vi "RecordSectionIMAQdx.vi"() -> ()   [LabVIEW 2009]
doc: "The Grab VI acquires images continuously and displays the images in an image control using high-level acquisition VIs. A grab is appropriate for high-speed applications in which you need to process only one image at a time."
uses:
  <vilib>/vision/driver/NI_Vision_Acquisition_Software.lvlib
  <vilib>/vision/Avi.llb/IMAQ AVI2 Refnum.ctl
panel:
  in  "Camera Name":refnum<k21> caption="IMAQdx Session"
  in  "Stop":bool
  out "Image":T1(plugin-control)
  in  "AVI File Path":path
  in  "Record":bool
  # "Overview: Demonstrates how to record a section of video while continuously using a Grab acquisition.  Can start and stop recording to specified AVI file path.\nRequirements: Vision Acquisition Software\nInstructions: \n1. Specify AVI File Path\n2. Select the Camera Interface.\n3. Run the VI\n4. Set Record booelean to true during segment of Grab you wish to record to AVI\n5. Set Recor boolean to false to end recording.\n6. Click Stop to terminate program."
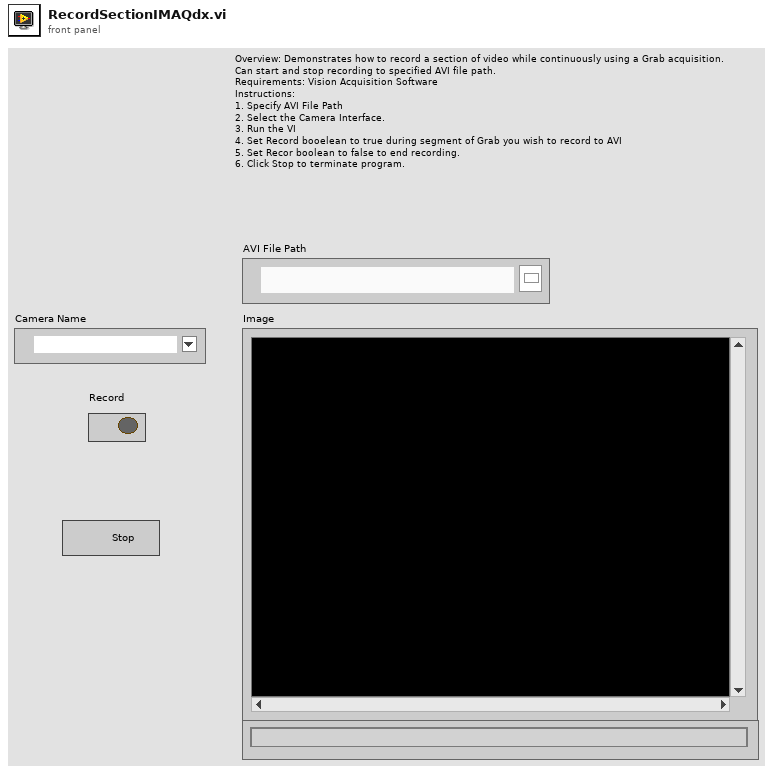
[diagram p1: front panel]
types:
  T1 = typedef "IMAQ Image.ctl" = refnum<image>
  T2 = typedef "Image Type" = u32
  T3 = typedef "IMAQdx.ctl" = refnum<k21>
  T4 = typedef "IMAQ AVI2 Refnum.ctl" = refnum<k20>
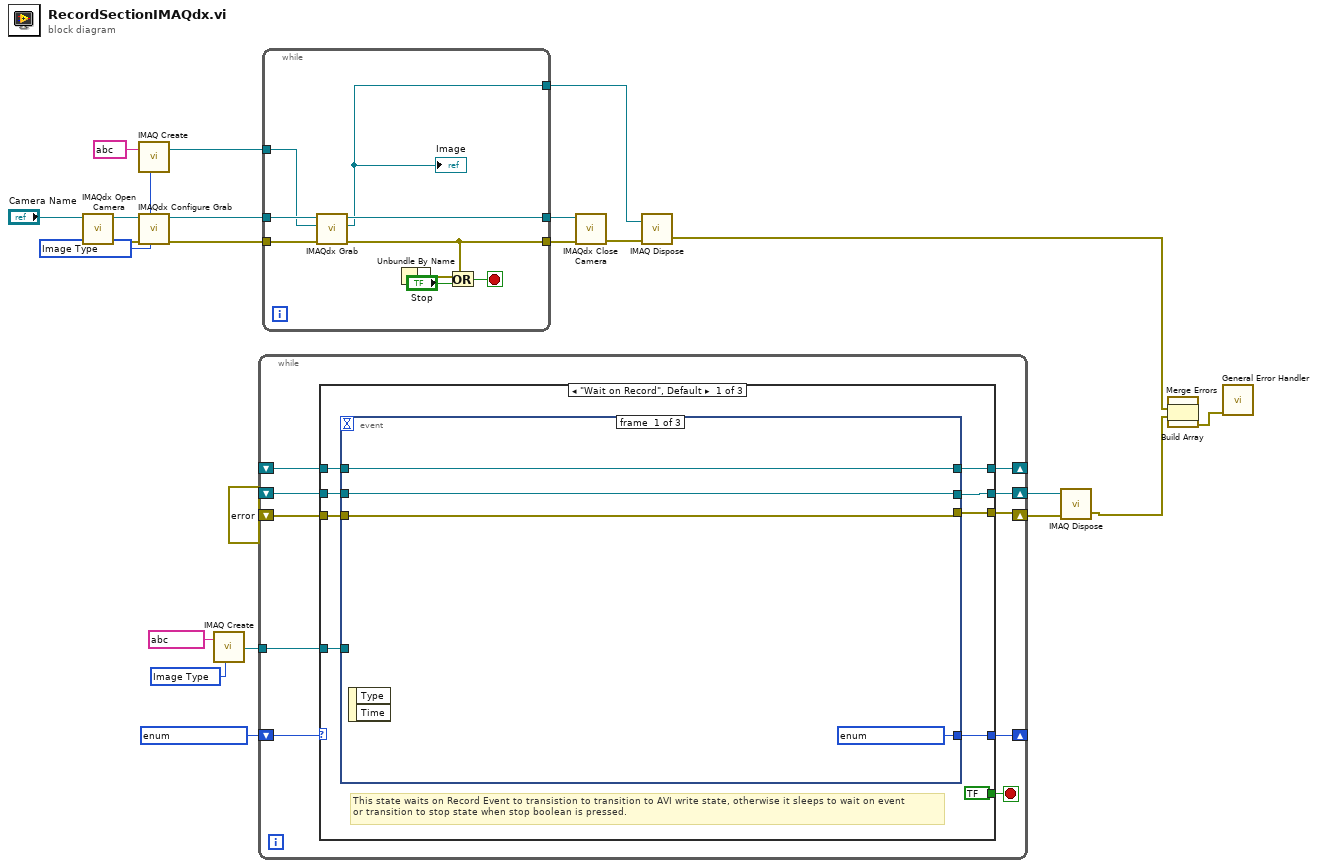
[diagram p0: block diagram]
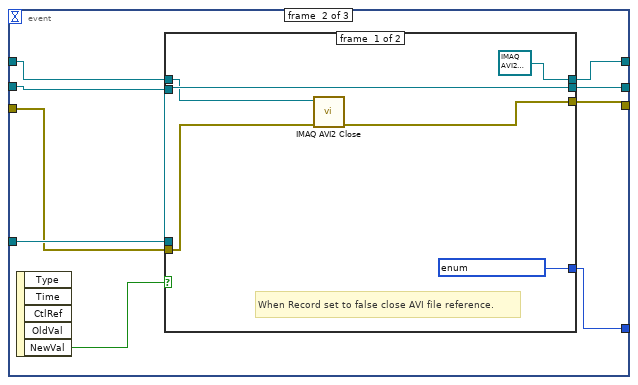
[diagram p2: hidden frame]
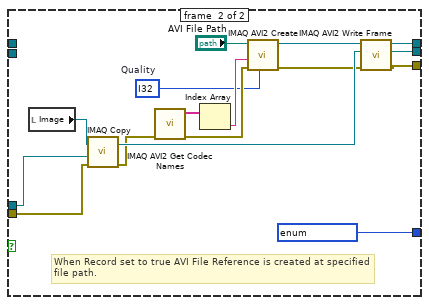
[diagram p3: hidden frame]
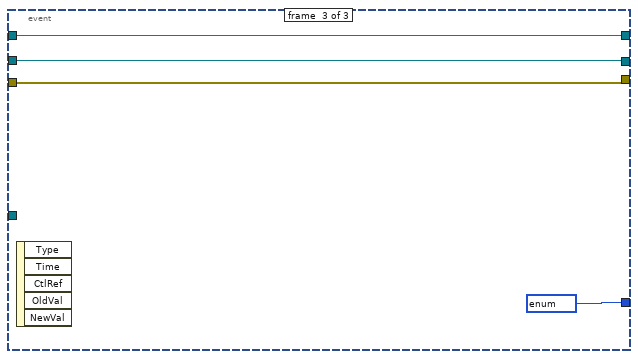
[diagram p4: hidden frame]
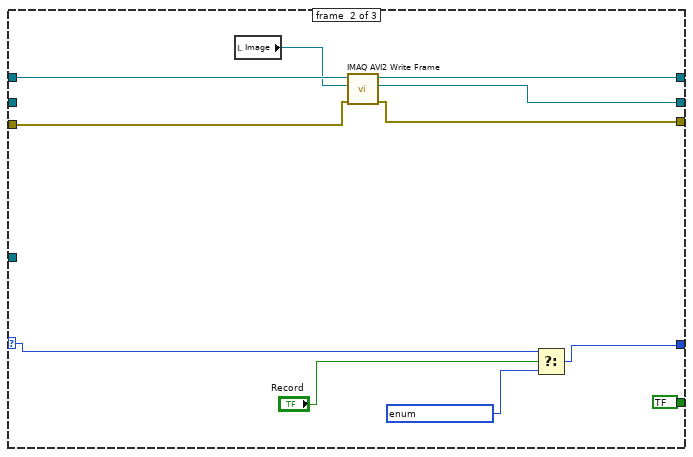
[diagram p5: hidden frame]
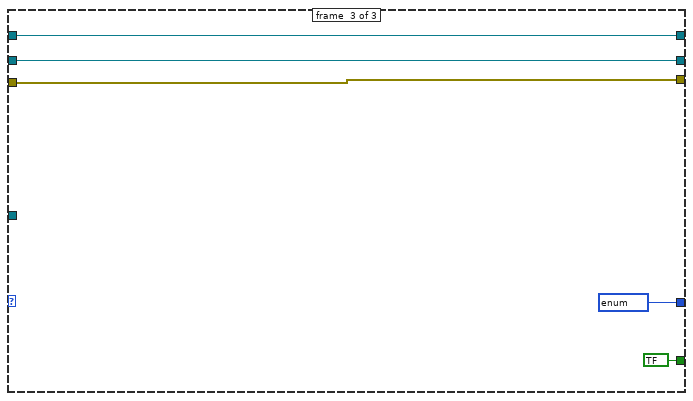
[diagram p6: hidden frame]
diagram:
  w2 = T2 ? items=["Grayscale (U8)", "Grayscale (I16)", "Grayscale (SGL)", "Complex (CSG)", "RGB (U32)", "HSL (U32)", "RGB (U64)", "Grayscale (U16)"] ("Image Type")
  w19 = T2 ? items=["Grayscale (U8)", "Grayscale (I16)", "Grayscale (SGL)", "Complex (CSG)", "RGB (U32)", "HSL (U32)", "RGB (U64)", "Grayscale (U16)"] ("Image Type")
  n1 = call <vilib>:"IMAQdx Open Camera.vi"("Session In"="Camera Name") -> ("error out"=w10:errorcluster, "Session Out"=w9:T3)  [unwired: 2 in, 7 out]
  n2 = call "IMAQ Create"("Image Name"=string ?, "Image Type"=w2) -> ("New Image"=w15:T1)  [unwired: 2 in, 2 out]
  n3 = call <vilib>:"IMAQdx Configure Grab.vi"("error in"=w10, "Session In"=w9) -> ("error out"=w13:errorcluster, "Session Out"=w14:T3)  [unwired: 8 out]
  n4 = call "IMAQ Create"("Image Name"=string ?, "Image Type"=w19) -> ("New Image"=w22:T1)  [unwired: 3 in, 1 out]
  n5 = while {
    tunnel: w22 -> [w33]
    shift-right: [w29] -> _
    shift-left: enum16{"Wait on Record", "Recording", "Stop"} ? -> [w30]
    shift-right: [w28] -> _
    shift-left: _ -> [w27]
    shift-right: [w31] -> w20
    shift-left: errorcluster ? ("error out") -> [w26]
    shift-right: [w32] -> w21
    shift-left: _ -> [w24]
    stop <- w25 stop-if-true
    n6 = case shown="\"Wait on Record\", Default" w30 {
      selector: w30 -> [_ w82 _]
      tunnel: w33 -> [w42 _ _]
      tunnel: [w41 w85 w93] -> w32
      tunnel: [w40 w88 w95] -> w31
      tunnel: [w39 w87 enum16{"Wait on Record", "Recording", "Stop"} ?] -> w29
      tunnel: [w38 w91 w96] -> w28
      tunnel: w27 -> [w37 w92 w96]
      tunnel: w26 -> [w36 w89 w95]
      tunnel: [bool ? bool ? bool ?] -> w25
      tunnel: w24 -> [w34 _ w93]
      frame #0 {
        # "This state waits on Record Event to transistion to transition to AVI write state, otherwise it sleeps to wait on event\nor transition to stop state when stop boolean is pressed."
        n7 = event shown="[1] \"Record\": Value Change" {
          selector: _ -> [_ _ _]
          dyn-events: _ -> [_ _ _]
          timeout: _ -> [_ _ _]
          tunnel: w42 -> [_ w55 _]
          tunnel: [w45 w54 w79] -> w41
          tunnel: [w46 w53 w78] -> w40
          tunnel: [enum16{"Wait on Record", "Recording", "Stop"} ? w47 enum16{"Wait on Record", "Recording", "Stop"} ?] -> w39
          tunnel: [w44 w52 w80] -> w38
          tunnel: w37 -> [w44 w50 w80]
          tunnel: w36 -> [w46 w51 w78]
          tunnel: w34 -> [w45 w49 w79]
          event #0 {
            n8 = event-data() -> ()  [unwired: 1 in, 2 out]
          }
          event #1 {
            n9 = event-data() -> ("NewVal"=w48:bool)  [unwired: 1 in, 4 out]
            n10 = case shown="True" w48 {
              tunnel: w55 -> [w61 w77]
              tunnel: [w61 w70] -> w54
              tunnel: [w57 w69] -> w53
              tunnel: [T4 ? ("AVI Refnum (duplicate)") w66] -> w52
              tunnel: w51 -> [w58 w63]
              tunnel: w50 -> [w59 _]
              tunnel: w49 -> [_ _]
              tunnel: [enum16{"Wait on Record", "Recording", "Stop"} ? enum16{"Wait on Record", "Recording", "Stop"} ?] -> w47
              frame #0 {
                # "When Record set to false close AVI file reference."
                n11 = call "IMAQ AVI2 Close"("error in (no error)"=w58, "AVI Refnum"=w59) -> ("error out"=w57:errorcluster)  [unwired: 9 in]
              }
              frame #1 {
                w73 = i32 ?  # Quality
                # "When Record set to true AVI File Reference is created at specified file path."
                n12 = local read "Image"() -> (w76:T1)
                n13 = call "IMAQ Copy"("error in (no error)"=w63, "Image Dst"=w77, "Image Src"=w76) -> ("error out"=w64:errorcluster, "Image Dst Out"=w68:T1)  [unwired: 3 in]
                n14 = call "IMAQ AVI2 Get Codec Names"("error in (no error)"=w64) -> ("error out"=w75:errorcluster, "Codec Names"=w72:string[])  [unwired: 9 in]
                n15 = Index Array(array=w72) -> (element=w74:string)  [unwired: 1 in]
                n16 = call "IMAQ AVI2 Create"("Quality"=w73, "error in (no error)"=w75, "Codec"=w74, "AVI Path"="AVI File Path") -> ("error out"=w65:errorcluster, "AVI Refnum"=w67:T4)  [unwired: 6 in]
                n17 = call "IMAQ AVI2 Write Frame"("error in (no error)"=w65, "Image"=w68, "AVI Refnum"=w67) -> ("error out"=w69:errorcluster, "Image Out (duplicate)"=w70:T1, "AVI Refnum (duplicate)"=w66:T4)  [unwired: 6 in]
              }
            }
          }
          event #2 {
            n18 = event-data() -> ()  [unwired: 1 in, 5 out]
          }
        }
      }
      frame #1 {
        n19 = local read "Image"() -> (w90:T1)
        n20 = call "IMAQ AVI2 Write Frame"("error in (no error)"=w89, "Image"=w90, "AVI Refnum"=w92) -> ("error out"=w88:errorcluster, "Image Out (duplicate)"=w85:T1, "AVI Refnum (duplicate)"=w91:T4)  [unwired: 6 in]
        n21 = Select(t=w82, s="Record", f=enum16{"Wait on Record", "Recording", "Stop"} ?) -> (s? t:f=w87:enum16{"Wait on Record", "Recording", "Stop"})
      }
      frame #2 {
      }
    }
  }
  n22 = while {
    tunnel: [w101] -> w12
    tunnel: w13 -> [w103]
    tunnel: w14 -> [w104]
    tunnel: [w100] -> w11
    tunnel: w15 -> [w102]
    tunnel: [w99] -> w7
    stop <- w106 stop-if-true
    n23 = call <vilib>:"IMAQdx Grab.vi"("error in"=w103, "Image In"=w102, "Session In"=w104) -> ("error out"=w100:errorcluster, "Image Out"=w99:T1, "Session Out"=w101:T3)  [unwired: 1 in, 5 out]
    "Image" <- w99
    n24 = Or(y="Stop") -> (x=w98:errorcluster, x .or. y?=w106:bool)
    n25 = Unbundle By Name(w100, w98) -> ()
  }
  n26 = call <vilib>:"IMAQdx Close Camera.vi"("error in"=w11, "Session In"=w12) -> ("error out"=w6:errorcluster)  [unwired: 9 out]
  n27 = call "IMAQ Dispose"("Image"=w7, "error in (no error)"=w6) -> ("error out"=w4:errorcluster)  [unwired: 4 in]
  n28 = call "IMAQ Dispose"("Image"=w21, "error in (no error)"=w20) -> ("error out"=w3:errorcluster)  [unwired: 1 in, 3 out]
  n29 = Build Array(w4, w3) -> (w1:errorcluster[])
  n30 = call <vilib>:"Merge Errors.vi"("error array in"=w1) -> ("error out"=w17:errorcluster)  [unwired: 6 in]
  n31 = call <vilib>:"General Error Handler.vi"("error in (no error)"=w17) -> ()  [unwired: 1 in, 14 out]
